vi "CR-SaveImage -CCD5NG.vi"(6 "CCD Name":string(combo), 8 "error in (no error)":errorcluster, 9 "Image in":T1(plugin-control), 10 "布尔":bool=TRUE, 11 "基路径":path) -> (0 "error out":errorcluster)   [LabVIEW 2017]
panel:
  out "连接的字符串":string
  # "D:\\Data\\History Image\\20190228\\CCD3\\Image"
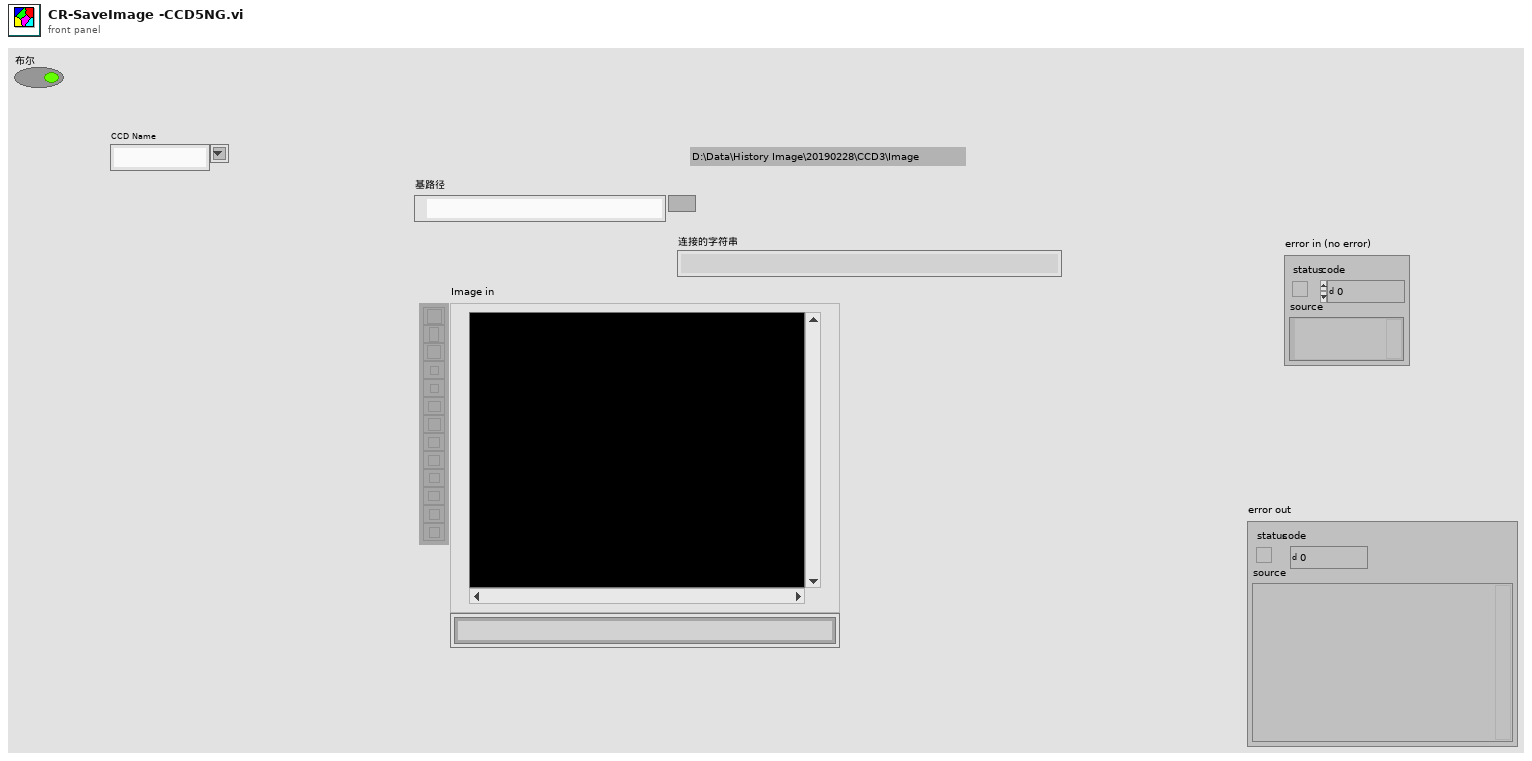
[diagram p1: front panel]
types:
  T1 = typedef "IMAQ Image.ctl" = refnum<image>
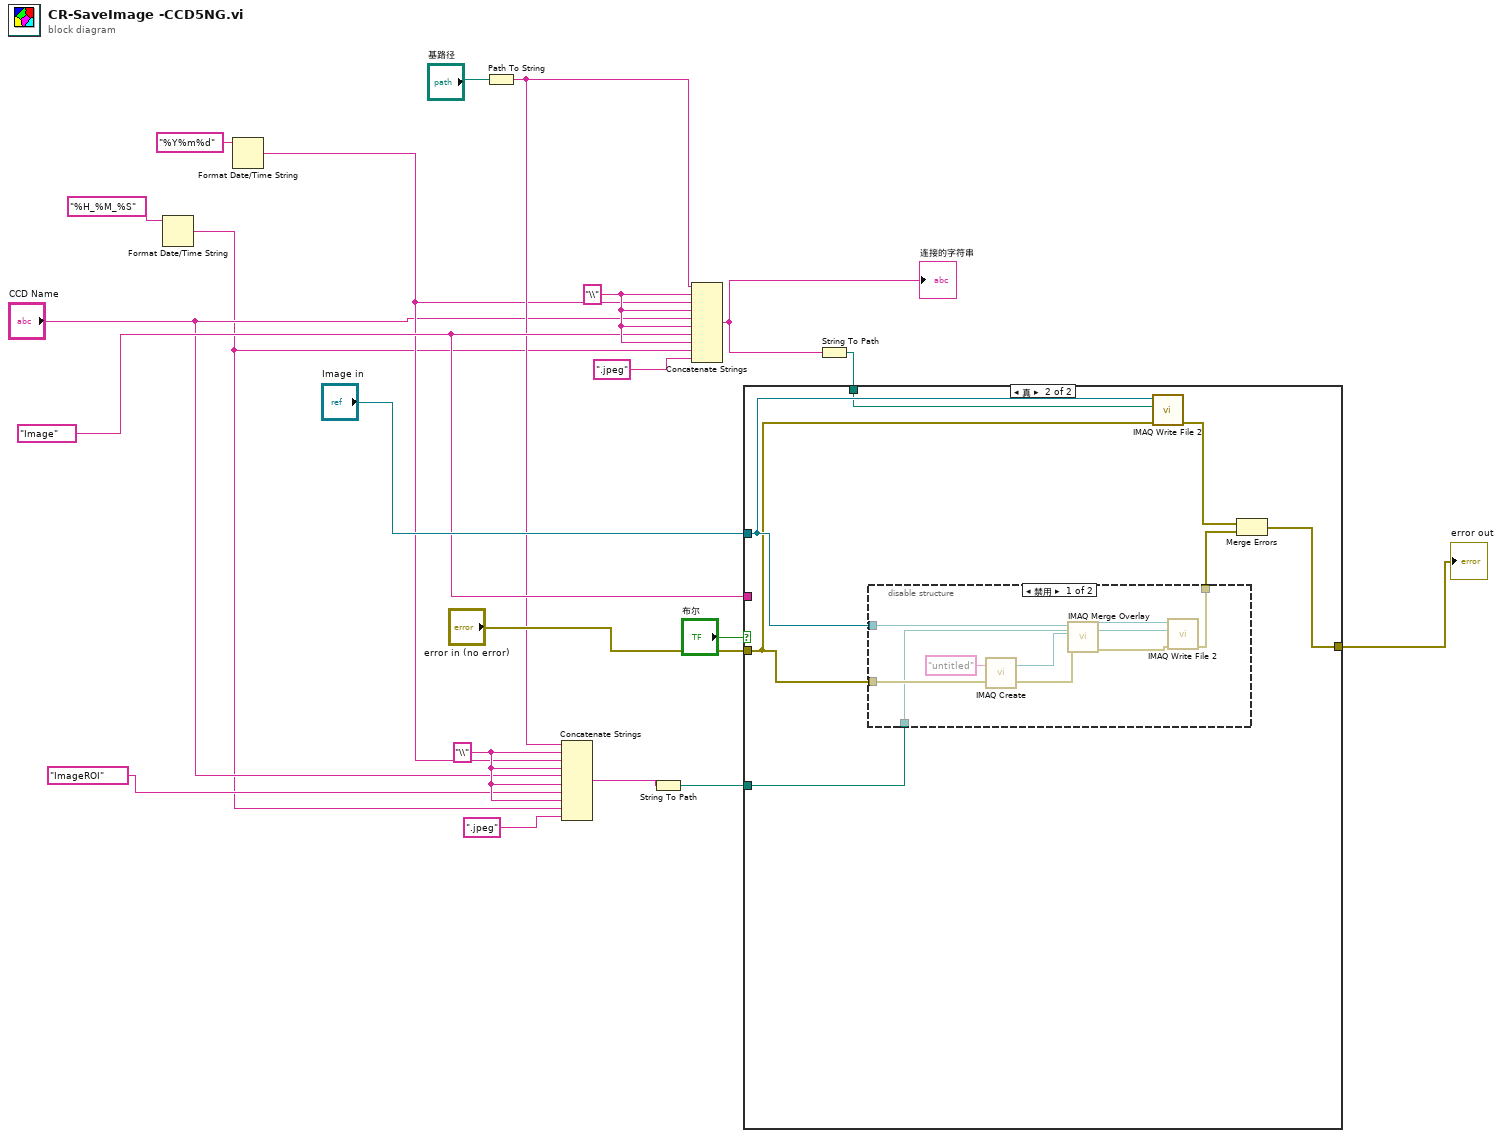
[diagram p0: block diagram]
diagram:
  w11 = "Image" ("类型")
  w9 = "\\" ("字符串")
  w13 = "\\" ("字符串")
  n1 = Format Date/Time String(time format string (%c)="%H_%M_%S" ("时间格式字符串(%c)")) -> (date/time string=w1:string)  [unwired: 2 in]
  n2 = Format Date/Time String(time format string (%c)="%Y%m%d" ("时间格式字符串(%c)")) -> (date/time string=w6:string)  [unwired: 2 in]
  n3 = Path To String(path="基路径") -> (string=w7:string)
  n4 = Concatenate Strings(w7, w9, w6, w9, "CCD Name", w9, "ImageROI" ("类型"), w9, w1, ".jpeg" ("字符串")) -> (w3:string)
  n5 = String To Path(string=w3) -> (path=w2:path)
  n6 = Concatenate Strings(w7, w13, w6, w13, "CCD Name", w13, w11, w13, w1, ".jpeg" ("字符串")) -> (w19:string)
  "连接的字符串" <- w19
  n7 = String To Path(string=w19) -> (path=w15:path)
  n8 = case shown="真" "布尔" {
    tunnel: "Image in" -> [_ w29]
    tunnel: "error in (no error)" -> [w22 w28]
    tunnel: w15 -> [_ w23]
    tunnel: [w22 w25] -> w12
    tunnel: w11 -> [_ _]
    tunnel: w2 -> [_ w24]
    frame False {
    }
    frame True {
      n9 = disable-structure shown="禁用" {
        disable-tunnel: w29 -> [w38 _]
        disable-tunnel: w28 -> [w37 _]
        disable-tunnel: [w31 _] -> w27
        disable-tunnel: w24 -> [w30 _]
        frame Disabled {
          n10 = call "IMAQ Create"("Image Name"="untitled", "error in (no error)"=w37) -> ("New Image"=w33:T1, "error out"=w32:errorcluster)  [unwired: 3 in]
          n11 = call "IMAQ Merge Overlay"("error in (no error)"=w32, "Image Dst"=w33, "Image Src"=w38) -> ("error out"=w35:errorcluster, "Image Dst Out"=w36:T1)  [unwired: 7 in]
          n12 = call-poly "IMAQ Write File 2"("error in (no error)"=w35, "File Path"=w30, "Image"=w36) -> ("error out"=w31:errorcluster)  [unwired: 7 in, 1 out]
        }
        frame Enabled {
        }
      }
      n13 = call-poly "IMAQ Write File 2"("error in (no error)"=w28, "File Path"=w23, "Image"=w29) -> ("error out"=w26:errorcluster)  [unwired: 7 in, 1 out]
      n14 = Merge Errors(w26, w27) -> (w25:errorcluster)
    }
  }
  "error out" <- w12
